vi "IndexOfNote.vi"(11 "Note":T1={"音名"=enum."A", "度"=enum."0", "變音記號"=enum.""}) -> (2 "名稱":string, 3 "index of note":i32)   [LabVIEW 2015]
uses:
  Note.ctl
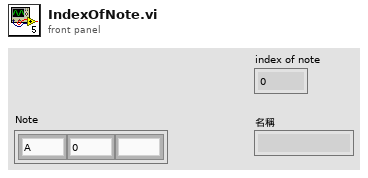
[diagram p1: front panel]
types:
  T1 = typedef "Note.ctl" = cluster{"音名":enum16{"C", "D", "E", "F", "G", "A", "B"}, "度":enum16{"0", "1", "2", "3", "4", "5", "6", "7", "8"}, "變音記號":enum16{"bb", "b", "", "#", "x"}}
  T2 = enum16{"0", "1", "2", "3", "4", "5", "6", "7", "8"}
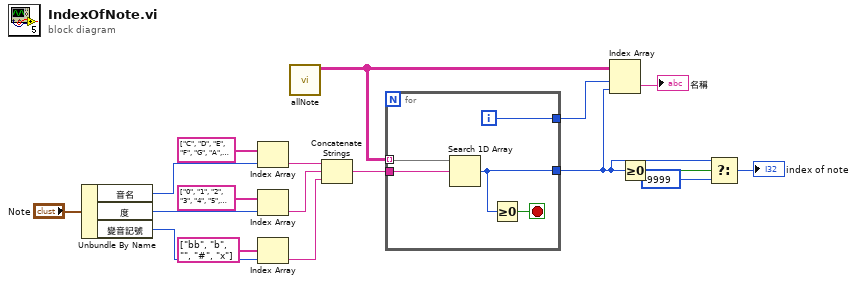
[diagram p0: block diagram]
diagram:
  n1 = Unbundle By Name("Note") -> ("音名"=w9:enum16{"C", "D", "E", "F", "G", "A", "B"}, "度"=w8:T2, "變音記號"=w7:enum16{"bb", "b", "", "#", "x"})
  n2 = Index Array(array=string[] ["C", "D", "E", "F", "G", "A", "B"], index=w9) -> (element=w15:string)
  n3 = Index Array(array=string[] ["0", "1", "2", "3", "4", "5", "6", "7", "8"], index=w8) -> (element=w14:string)
  n4 = Index Array(array=string[] ["bb", "b", "", "#", "x"], index=w7) -> (element=w13:string)
  n5 = call "allNote.vi"() -> ("Allnote"=w2:string[][])  [unwired: 10 in, 1 out]
  n6 = Concatenate Strings(w15, w14, w13) -> (w11:string)
  n7 = for {
    tunnel: w2 -> [w23] mode=indexing
    tunnel: w11 -> [w22]
    tunnel: [w20] -> w4
    tunnel: [w19] -> w12
    i -> [w19]
    stop <- w21 stop-if-true
    n8 = Search 1D Array(1D array=w23, element=w22) -> (index of element=w20:i32)  [unwired: 1 in]
    n9 = Greater Or Equal To 0?(x=w20) -> (x >= 0?=w21:bool)
  }
  n10 = Index Array(array=w2, index (row)=w12, index (col)=w4) -> (element=→"名稱":string)
  n11 = Greater Or Equal To 0?(x=w4) -> (x >= 0?=w6:bool)
  n12 = Select(t=w4, s=w6, f=-9999) -> (s? t:f=→"index of note":i32)
